vi "GeoData.vi"() -> ()   [LabVIEW 2017] (continued)
98357\t53009\tNeah bay\tWA\tClallam County\tH1\n98331\t53009\tForks\tWA\tClallam County\tH1\n98362\t53009\tPort angeles\tWA\tClallam County\tH1\n98343\t53009\tJoyce\tWA\tClallam County\tH1\n98350\t53009\tLa push\tWA\tClallam County\tH1\n98606\t53011\tBrush prairie\tWA\tClark County\tH1\n98601\t53011\tAmboy\tWA\tClark County\tH1\n98671\t53011\tWashougal\tWA\tClark County\tH1\n98674\t53011\tWoodland\tWA\tClark County\tH1\n98682\t53011\tVancouver\tWA\tClark County\tH1\n98668\t53011\tVancouver\tWA\tClark County\tH1\n98607\t53011\tCamas\tWA\tClark County\tH1\n98662\t53011\tVancouver\tWA\tClark County\tH1\n98687\t53011\tVancouver\tWA\tClark County\tH1\n98604\t53011\tBattle ground\tWA\tClark County\tH1\n98642\t53011\tRidgefield\tWA\tClark County\tH1\n98629\t53011\tLa center\tWA\tClark County\tH1\n98663\t53011\tVancouver\tWA\tClark County\tH1\n98685\t53011\tVancouver\tWA\tClark County\tH1\n98622\t53011\tHeisson\tWA\tClark County\tH1\n98664\t53011\tVancouver\tWA\tClark County\tH1\n98686\t53011\tVancouver\tWA\tClark County\tH1\n98660\t53011\tVancouver\tWA\tClark County\tH1\n98683\t53011\tVancouver\tWA\tClark County\tH1\n98665\t53011\tVancouver\tWA\tClark County\tH1\n98684\t53011\tVancouver\tWA\tClark County\tH1\n98675\t53011\tYacolt\tWA\tClark County\tH1\n98666\t53011\tVancouver\tWA\tClark County\tH1\n98661\t53011\tVancouver\tWA\tClark County\tH1\n99328\t53013\tDayton\tWA\tColumbia County\tH1\n99361\t53013\tWaitsburg\tWA\tColumbia County\tH1\n99359\t53013\tStarbuck\tWA\tColumbia County\tH1\n99347\t53013\tPomeroy\tWA\tColumbia County\tH1\n99348\t53013\tPrescott\tWA\tColumbia County\tH1\n99143\t53013\tLacrosse\tWA\tColumbia County\tH1\n98601\t53015\tAmboy\tWA\tCowlitz County\tH1\n98674\t53015\tWoodland\tWA\tCowlitz County\tH1\n98581\t53015\tRyderwood\tWA\tCowlitz County\tH1\n98609\t53015\tCarrolls\tWA\tCowlitz County\tH1\n98649\t53015\tToutle\tWA\tCowlitz County\tH1\n98611\t53015\tCastle rock\tWA\tCowlitz County\tH1\n98625\t53015\tKalama\tWA\tCowlitz County\tH1\n98645\t53015\tSilverlake\tWA\tCowlitz County\tH1\n98616\t53015\tCougar\tWA\tCowlitz County\tH1\n98632\t53015\tLongview\tWA\tCowlitz County\tH1\n98603\t53015\tAriel\tWA\tCowlitz County\tH1\n98626\t53015\tKelso\tWA\tCowlitz County\tH1\n98858\t53017\tWaterville\tWA\tDouglas County\tH1\n98845\t53017\tPalisades\tWA\tDouglas County\tH1\n98848\t53017\tQuincy\tWA\tDouglas County\tH1\n98830\t53017\tMansfield\tWA\tDouglas County\tH1\n98802\t53017\tEast wenatchee\tWA\tDouglas County\tH1\n99133\t53017\tGrand coulee\tWA\tDouglas County\tH1\n98823\t53017\tEphrata\tWA\tDouglas County\tH1\n98843\t53017\tOrondo\tWA\tDouglas County\tH1\n98850\t53017\tRock island\tWA\tDouglas County\tH1\n98812\t53017\tBrewster\tWA\tDouglas County\tH1\n99115\t53017\tCoulee city\tWA\tDouglas County\tH1\n99116\t53017\tCoulee dam\tWA\tDouglas County\tH1\n98813\t53017\tBridgeport\tWA\tDouglas County\tH1\n99121\t53019\tDanville\tWA\tFerry County\tH1\n99166\t53019\tRepublic\tWA\tFerry County\tH1\n99118\t53019\tCurlew\tWA\tFerry County\tH1\n99141\t53019\tKettle falls\tWA\tFerry County\tH1\n99146\t53019\tLaurier\tWA\tFerry County\tH1\n99140\t53019\tKeller\tWA\tFerry County\tH1\n99138\t53019\tInchelium\tWA\tFerry County\tH1\n99150\t53019\tMalo\tWA\tFerry County\tH1\n99160\t53019\tOrient\tWA\tFerry County\tH1\n99330\t53021\tEltopia\tWA\tFranklin County\tH1\n99371\t53021\tWashtucna\tWA\tFranklin County\tH1\n99335\t53021\tKahlotus\tWA\tFranklin County\tH1\n99343\t53021\tMesa\tWA\tFranklin County\tH1\n99344\t53021\tOthello\tWA\tFranklin County\tH1\n99302\t53021\tPasco\tWA\tFranklin County\tH1\n99301\t53021\tPasco\tWA\tFranklin County\tH1\n99326\t53021\tConnell\tWA\tFranklin County\tH1\n99328\t53023\tDayton\tWA\tGarfield County\tH1\n99347\t53023\tPomeroy\tWA\tGarfield County\tH1\n99403\t53023\tClarkston\tWA\tGarfield County\tH1\n98857\t53025\tWarden\tWA\tGrant County\tH1\n99357\t53025\tRoyal city\tWA\tGrant County\tH1\n98858\t53025\tWaterville\tWA\tGrant County\tH1\n98860\t53025\tWilson creek\tWA\tGrant County\tH1\n98851\t53025\tSoap lake\tWA\tGrant County\tH1\n99103\t53025\tAlmira\tWA\tGrant County\tH1\n98824\t53025\tGeorge\tWA\tGrant County\tH1\n98848\t53025\tQuincy\tWA\tGrant County\tH1\n99349\t53025\tMattawa\tWA\tGrant County\tH1\n98853\t53025\tStratford\tWA\tGrant County\tH1\n99133\t53025\tGrand coulee\tWA\tGrant County\tH1\n99123\t53025\tElectric city\tWA\tGrant County\tH1\n99344\t53025\tOthello\tWA\tGrant County\tH1\n99321\t53025\tBeverly\tWA\tGrant County\tH1\n98832\t53025\tMarlin\tWA\tGrant County\tH1\n98823\t53025\tEphrata\tWA\tGrant County\tH1\n99135\t53025\tHartline\tWA\tGrant County\tH1\n98837\t53025\tMoses lake\tWA\tGrant County\tH1\n99115\t53025\tCoulee city\tWA\tGrant County\tH1\n99116\t53025\tCoulee dam\tWA\tGrant County\tH1\n98537\t53027\tCosmopolis\tWA\tGrays Harbor County\tH1\n98563\t53027\tMontesano\tWA\tGrays Harbor County\tH1\n98595\t53027\tWestport\tWA\tGrays Harbor County\tH1\n98550\t53027\tHoquiam\tWA\tGrays Harbor County\tH1\n98583\t53027\tSatsop\tWA\tGrays Harbor County\tH1\n98569\t53027\tOcean shores\tWA\tGrays Harbor County\tH1\n98520\t53027\tAberdeen\tWA\tGrays Harbor County\tH1\n98526\t53027\tAmanda park\tWA\tGrays Harbor County\tH1\n98575\t53027\tQuinault\tWA\tGrays Harbor County\tH1\n98562\t53027\tMoclips\tWA\tGrays Harbor County\tH1\n98557\t53027\tMccleary\tWA\tGrays Harbor County\tH1\n98579\t53027\tRochester\tWA\tGrays Harbor County\tH1\n98541\t53027\tElma\tWA\tGrays Harbor County\tH1\n98547\t53027\tGrayland\tWA\tGrays Harbor County\tH1\n98568\t53027\tOakville\tWA\tGrays Harbor County\tH1\n98536\t53027\tCopalis crossing\tWA\tGrays Harbor County\tH1\n98566\t53027\tNeilton\tWA\tGrays Harbor County\tH1\n98535\t53027\tCopalis beach\tWA\tGrays Harbor County\tH1\n98571\t53027\tPacific beach\tWA\tGrays Harbor County\tH1\n98552\t53027\tHumptulips\tWA\tGrays Harbor County\tH1\n98559\t53027\tMalone\tWA\tGrays Harbor County\tH1\n98587\t53027\tTaholah\tWA\tGrays Harbor County\tH1\n98249\t53029\tFreeland\tWA\tIsland County\tH1\n98278\t53029\tOak harbor\tWA\tIsland County\tH1\n98277\t53029\tOak harbor\tWA\tIsland County\tH1\n98282\t53029\tCamano island\tWA\tIsland County\tH1\n98260\t53029\tLangley\tWA\tIsland County\tH1\n98236\t53029\tClinton\tWA\tIsland County\tH1\n98253\t53029\tGreenbank\tWA\tIsland County\tH1\n98239\t53029\tCoupeville\tWA\tIsland County\tH1\n98320\t53031\tBrinnon\tWA\tJefferson County\tH1\n98376\t53031\tQuilcene\tWA\tJefferson County\tH1\n98368\t53031\tPort townsend\tWA\tJefferson County\tH1\n98365\t53031\tPort ludlow\tWA\tJefferson County\tH1\n98382\t53031\tSequim\tWA\tJefferson County\tH1\n98331\t53031\tForks\tWA\tJefferson County\tH1\n98339\t53031\tPort hadlock\tWA\tJefferson County\tH1\n98325\t53031\tChimacum\tWA\tJefferson County\tH1\n98358\t53031\tNordland\tWA\tJefferson County\tH1\n98102\t53033\tSeattle\tWA\tKing County\tH1\n98103\t53033\tSeattle\tWA\tKing County\tH1\n98115\t53033\tSeattle\tWA\tKing County\tH1\n98058\t53033\tRenton\tWA\tKing County\tH1\n98070\t53033\tVashon\tWA\tKing County\tH1\n98122\t53033\tSeattle\tWA\tKing County\tH1\n98083\t53033\tKirkland\tWA\tKing County\tH1\n98111\t53033\tSeattle\tWA\tKing County\tH1\n98198\t53033\tSeattle\tWA\tKing County\tH1\n98133\t53033\tSeattle\tWA\tKing County\tH1\n98136\t53033\tSeattle\tWA\tKing County\tH1\n98134\t53033\tSeattle\tWA\tKing County\tH1\n98034\t53033\tKirkland\tWA\tKing County\tH1\n98023\t53033\tFederal way\tWA\tKing County\tH1\n98052\t53033\tRedmond\tWA\tKing County\tH1\n98021\t53033\tBothell\tWA\tKing County\tH1\n98055\t53033\tRenton\tWA\tKing County\tH1\n98051\t53033\tRavensdale\tWA\tKing County\tH1\n98194\t53033\tSeattle\tWA\tKing County\tH1\n98175\t53033\tSeattle\tWA\tKing County\tH1\n98224\t53033\tBaring\tWA\tKing County\tH1\n98004\t53033\tBellevue\tWA\tKing County\tH1\n98007\t53033\tBellevue\tWA\tKing County\tH1\n98008\t53033\tBellevue\tWA\tKing County\tH1\n98019\t53033\tDuvall\tWA\tKing County\tH1\n98014\t53033\tCarnation\tWA\tKing County\tH1\n98092\t53033\tAuburn\tWA\tKing County\tH1\n98074\t53033\tSammamish\tWA\tKing County\tH1\n98106\t53033\tSeattle\tWA\tKing County\tH1\n98354\t53033\tMilton\tWA\tKing County\tH1\n98030\t53033\tKent\tWA\tKing County\tH1\n98288\t53033\tSkykomish\tWA\tKing County\tH1\n98035\t53033\tKent\tWA\tKing County\tH1\n98131\t53033\tSeattle\tWA\tKing County\tH1\n98001\t53033\tAuburn\tWA\tKing County\tH1\n98119\t53033\tSeattle\tWA\tKing County\tH1\n98144\t53033\tSeattle\tWA\tKing County\tH1\n98126\t53033\tSeattle\tWA\tKing County\tH1\n98124\t53033\tSeattle\tWA\tKing County\tH1\n98042\t53033\tKent\tWA\tKing County\tH1\n98158\t53033\tSeattle\tWA\tKing County\tH1\n98073\t53033\tRedmond\tWA\tKing County\tH1\n98113\t53033\tSeattle\tWA\tKing County\tH1\n98071\t53033\tAuburn\tWA\tKing County\tH1\n98062\t53033\tSeahurst\tWA\tKing County\tH1\n98129\t53033\tSeattle\tWA\tKing County\tH1\n98002\t53033\tAuburn\tWA\tKing County\tH1\n98011\t53033\tBothell\tWA\tKing County\tH1\n98006\t53033\tBellevue\tWA\tKing County\tH1\n98188\t53033\tSeattle\tWA\tKing County\tH1\n98199\t53033\tSeattle\tWA\tKing County\tH1\n98031\t53033\tKent\tWA\tKing County\tH1\n98022\t53033\tEnumclaw\tWA\tKing County\tH1\n98033\t53033\tKirkland\tWA\tKing County\tH1\n98039\t53033\tMedina\tWA\tKing County\tH1\n98057\t53033\tRenton\tWA\tKing County\tH1\n98045\t53033\tNorth bend\tWA\tKing County\tH1\n98089\t53033\tKent\tWA\tKing County\tH1\n98063\t53033\tFederal way\tWA\tKing County\tH1\n98025\t53033\tHobart\tWA\tKing County\tH1\n98191\t53033\tSeattle\tWA\tKing County\tH1\n98003\t53033\tFederal way\tWA\tKing County\tH1\n98109\t53033\tSeattle\tWA\tKing County\tH1\n98117\t53033\tSeattle\tWA\tKing County\tH1\n98118\t53033\tSeattle\tWA\tKing County\tH1\n98121\t53033\tSeattle\tWA\tKing County\tH1\n98155\t53033\tSeattle\tWA\tKing County\tH1\n98038\t53033\tMaple valley\tWA\tKing County\tH1\n98032\t53033\tKent\tWA\tKing County\tH1\n98024\t53033\tFall city\tWA\tKing County\tH1\n98053\t53033\tRedmond\tWA\tKing County\tH1\n98138\t53033\tSeattle\tWA\tKing County\tH1\n98181\t53033\tSeattle\tWA\tKing County\tH1\n98010\t53033\tBlack diamond\tWA\tKing County\tH1\n98107\t53033\tSeattle\tWA\tKing County\tH1\n98065\t53033\tSnoqualmie\tWA\tKing County\tH1\n98072\t53033\tWoodinville\tWA\tKing County\tH1\n98112\t53033\tSeattle\tWA\tKing County\tH1\n98146\t53033\tSeattle\tWA\tKing County\tH1\n98148\t53033\tSeattle\tWA\tKing County\tH1\n98145\t53033\tSeattle\tWA\tKing County\tH1\n98185\t53033\tSeattle\tWA\tKing County\tH1\n98050\t53033\tPreston\tWA\tKing County\tH1\n98009\t53033\tBellevue\tWA\tKing County\tH1\n98101\t53033\tSeattle\tWA\tKing County\tH1\n98108\t53033\tSeattle\tWA\tKing County\tH1\n98077\t53033\tWoodinville\tWA\tKing County\tH1\n98093\t53033\tFederal way\tWA\tKing County\tH1\n98251\t53033\tGold bar\tWA\tKing County\tH1\n98422\t53033\tTacoma\tWA\tKing County\tH1\n98168\t53033\tSeattle\tWA\tKing County\tH1\n98177\t53033\tSeattle\tWA\tKing County\tH1\n98125\t53033\tSeattle\tWA\tKing County\tH1\n98178\t53033\tSeattle\tWA\tKing County\tH1\n98127\t53033\tSeattle\tWA\tKing County\tH1\n98028\t53033\tKenmore\tWA\tKing County\tH1\n98047\t53033\tPacific\tWA\tKing County\tH1\n98164\t53033\tSeattle\tWA\tKing County\tH1\n98015\t53033\tBellevue\tWA\tKing County\tH1\n98154\t53033\tSeattle\tWA\tKing County\tH1\n98195\t53033\tSeattle\tWA\tKing County\tH1\n98068\t53033\tSnoqualmie pass\tWA\tKing County\tH1\n98005\t53033\tBellevue\tWA\tKing County\tH1\n98104\t53033\tSeattle\tWA\tKing County\tH1\n98105\t53033\tSeattle\tWA\tKing County\tH1\n98059\t53033\tRenton\tWA\tKing County\tH1\n98075\t53033\tSammamish\tWA\tKing County\tH1\n98116\t53033\tSeattle\tWA\tKing County\tH1\n98166\t53033\tSeattle\tWA\tKing County\tH1\n98029\t53033\tIssaquah\tWA\tKing County\tH1\n98040\t53033\tMercer island\tWA\tKing County\tH1\n98027\t53033\tIssaquah\tWA\tKing County\tH1\n98056\t53033\tRenton\tWA\tKing County\tH1\n98165\t53033\tSeattle\tWA\tKing County\tH1\n98041\t53033\tBothell\tWA\tKing County\tH1\n98139\t53033\tSeattle\tWA\tKing County\tH1\n98174\t53033\tSeattle\tWA\tKing County\tH1\n98064\t53033\tKent\tWA\tKing County\tH1\n98161\t53033\tSeattle\tWA\tKing County\tH1\n98114\t53033\tSeattle\tWA\tKing County\tH1\n98359\t53035\tOlalla\tWA\tKitsap County\tH1\n98353\t53035\tManchester\tWA\tKitsap County\tH1\n98312\t53035\tBremerton\tWA\tKitsap County\tH1\n98329\t53035\tGig harbor\tWA\tKitsap County\tH1\n98380\t53035\tSeabeck\tWA\tKitsap County\tH1\n98342\t53035\tIndianola\tWA\tKitsap County\tH1\n98340\t53035\tHansville\tWA\tKitsap County\tH1\n98364\t53035\tPort gamble\tWA\tKitsap County\tH1\n98366\t53035\tPort orchard\tWA\tKitsap County\tH1\n98110\t53035\tBainbridge island\tWA\tKitsap County\tH1\n98370\t53035\tPoulsbo\tWA\tKitsap County\tH1\n98346\t53035\tKingston\tWA\tKitsap County\tH1\n98322\t53035\tBurley\tWA\tKitsap County\tH1\n98384\t53035\tSouth colby\tWA\tKitsap County\tH1\n98315\t53035\tSilverdale\tWA\tKitsap County\tH1\n98392\t53035\tSuquamish\tWA\tKitsap County\tH1\n98393\t53035\tTracyton\tWA\tKitsap County\tH1\n98345\t53035\tKeyport\tWA\tKitsap County\tH1\n98061\t53035\tRollingbay\tWA\tKitsap County\tH1\n98311\t53035\tBremerton\tWA\tKitsap County\tH1\n98310\t53035\tBremerton\tWA\tKitsap County\tH1\n98367\t53035\tPort orchard\tWA\tKitsap County\tH1\n98337\t53035\tBremerton\tWA\tKitsap County\tH1\n98314\t53035\tBremerton\tWA\tKitsap County\tH1\n98383\t53035\tSilverdale\tWA\tKitsap County\tH1\n98528\t53035\tBelfair\tWA\tKitsap County\tH1\n98386\t53035\tSouthworth\tWA\tKitsap County\tH1\n98828\t53037\tMalaga\tWA\tKittitas County\tH1\n98941\t53037\tRoslyn\tWA\tKittitas County\tH1\n98922\t53037\tCle elum\tWA\tKittitas County\tH1\n98926\t53037\tEllensburg\tWA\tKittitas County\tH1\n98943\t53037\tSouth cle elum\tWA\tKittitas County\tH1\n98950\t53037\tVantage\tWA\tKittitas County\tH1\n98901\t53037\tYakima\tWA\tKittitas County\tH1\n98946\t53037\tThorp\tWA\tKittitas County\tH1\n98925\t53037\tEaston\tWA\tKittitas County\tH1\n98812\t53037\tBrewster\tWA\tKittitas County\tH1\n98940\t53037\tRonald\tWA\tKittitas County\tH1\n98068\t53037\tSnoqualmie pass\tWA\tKittitas County\tH1\n98934\t53037\tKittitas\tWA\tKittitas County\tH1\n98623\t53039\tHusum\tWA\tKlickitat County\tH1\n98617\t53039\tDallesport\tWA\tKlickitat County\tH1\n99356\t53039\tRoosevelt\tWA\tKlickitat County\tH1\n99322\t53039\tBickleton\tWA\tKlickitat County\tH1\n98620\t53039\tGoldendale\tWA\tKlickitat County\tH1\n98605\t53039\tBingen\tWA\tKlickitat County\tH1\n98673\t53039\tWishram\tWA\tKlickitat County\tH1\n98650\t53039\tTrout lake\tWA\tKlickitat County\tH1\n98635\t53039\tLyle\tWA\tKlickitat County\tH1\n99350\t53039\tProsser\tWA\tKlickitat County\tH1\n98602\t53039\tAppleton\tWA\tKlickitat County\tH1\n98935\t53039\tMabton\tWA\tKlickitat County\tH1\n98651\t53039\tUnderwood\tWA\tKlickitat County\tH1\n98619\t53039\tGlenwood\tWA\tKlickitat County\tH1\n98628\t53039\tKlickitat\tWA\tKlickitat County\tH1\n98672\t53039\tWhite salmon\tWA\tKlickitat County\tH1\n98613\t53039\tCenterville\tWA\tKlickitat County\tH1\n98670\t53039\tWahkiacus\tWA\tKlickitat County\tH1\n98539\t53041\tDoty\tWA\tLewis County\tH1\n98330\t53041\tElbe\tWA\tLewis County\tH1\n98355\t53041\tMineral\tWA\tLewis County\tH1\n98532\t53041\tChehalis\tWA\tLewis County\tH1\n98572\t53041\tPe ell\tWA\tLewis County\tH1\n98538\t53041\tCurtis\tWA\tLewis County\tH1\n98582\t53041\tSalkum\tWA\tLewis County\tH1\n98377\t53041\tRandle\tWA\tLewis County\tH1\n98533\t53041\tCinebar\tWA\tLewis County\tH1\n98579\t53041\tRochester\tWA\tLewis County\tH1\n98591\t53041\tToledo\tWA\tLewis County\tH1\n98542\t53041\tEthel\tWA\tLewis County\tH1\n98304\t53041\tAshford\tWA\tLewis County\tH1\n98531\t53041\tCentralia\tWA\tLewis County\tH1\n98596\t53041\tWinlock\tWA\tLewis County\tH1\n98361\t53041\tPackwood\tWA\tLewis County\tH1\n98593\t53041\tVader\tWA\tLewis County\tH1\n98522\t53041\tAdna\tWA\tLewis County\tH1\n98544\t53041\tGalvin\tWA\tLewis County\tH1\n98570\t53041\tOnalaska\tWA\tLewis County\tH1\n98568\t53041\tOakville\tWA\tLewis County\tH1\n98585\t53041\tSilver creek\tWA\tLewis County\tH1\n98336\t53041\tGlenoma\tWA\tLewis County\tH1\n98356\t53041\tMorton\tWA\tLewis County\tH1\n98564\t53041\tMossyrock\tWA\tLewis County\tH1\n98565\t53041\tNapavine\tWA\tLewis County\tH1\n99032\t53043\tSprague\tWA\tLincoln County\tH1\n99154\t53043\tMohler\tWA\tLincoln County\tH1\n99144\t53043\tLamona\tWA\tLincoln County\tH1\n99185\t53043\tWilbur\tWA\tLincoln County\tH1\n99103\t53043\tAlmira\tWA\tLincoln County\tH1\n99147\t53043\tLincoln\tWA\tLincoln County\tH1\n99169\t53043\tRitzville\tWA\tLincoln County\tH1\n99133\t53043\tGrand coulee\tWA\tLincoln County\tH1\n99029\t53043\tReardan\tWA\tLincoln County\tH1\n99134\t53043\tHarrington\tWA\tLincoln County\tH1\n99122\t53043\tDavenport\tWA\tLincoln County\tH1\n98832\t53043\tMarlin\tWA\tLincoln County\tH1\n99008\t53043\tEdwall\tWA\tLincoln County\tH1\n99159\t53043\tOdessa\tWA\tLincoln County\tH1\n99117\t53043\tCreston\tWA\tLincoln County\tH1\n99013\t53043\tFord\tWA\tLincoln County\tH1\n98563\t53045\tMontesano\tWA\tMason County\tH1\n98312\t53045\tBremerton\tWA\tMason County\tH1\n98380\t53045\tSeabeck\tWA\tMason County\tH1\n98592\t53045\tUnion\tWA\tMason County\tH1\n98560\t53045\tMatlock\tWA\tMason County\tH1\n98502\t53045\tOlympia\tWA\tMason County\tH1\n98557\t53045\tMccleary\tWA\tMason County\tH1\n98524\t53045\tAllyn\tWA\tMason County\tH1\n98541\t53045\tElma\tWA\tMason County\tH1\n98584\t53045\tShelton\tWA\tMason County\tH1\n98588\t53045\tTahuya\tWA\tMason County\tH1\n98555\t53045\tLilliwaup\tWA\tMason County\tH1\n98548\t53045\tHoodsport\tWA\tMason County\tH1\n98528\t53045\tBelfair\tWA\tMason County\tH1\n98546\t53045\tGrapeview\tWA\tMason County\tH1\n98862\t53047\tWinthrop\tWA\tOkanogan County\tH1\n99124\t53047\tElmer city\tWA\tOkanogan County\tH1\n98816\t53047\tChelan\tWA\tOkanogan County\tH1\n98814\t53047\tCarlton\tWA\tOkanogan County\tH1\n99166\t53047\tRepublic\tWA\tOkanogan County\tH1\n98846\t53047\tPateros\tWA\tOkanogan County\tH1\n98819\t53047\tConconully\tWA\tOkanogan County\tH1\n98849\t53047\tRiverside\tWA\tOkanogan County\tH1\n98834\t53047\tMethow\tWA\tOkanogan County\tH1\n98844\t53047\tOroville\tWA\tOkanogan County\tH1\n99133\t53047\tGrand coulee\tWA\tOkanogan County\tH1\n98841\t53047\tOmak\tWA\tOkanogan County\tH1\n98833\t53047\tMazama\tWA\tOkanogan County\tH1\n98855\t53047\tTonasket\tWA\tOkanogan County\tH1\n98840\t53047\tOkanogan\tWA\tOkanogan County\tH1\n98812\t53047\tBrewster\tWA\tOkanogan County\tH1\n98859\t53047\tWauconda\tWA\tOkanogan County\tH1\n98856\t53047\tTwisp\tWA\tOkanogan County\tH1\n99155\t53047\tNespelem\tWA\tOkanogan County\tH1\n98827\t53047\tLoomis\tWA\tOkanogan County\tH1\n99116\t53047\tCoulee dam\tWA\tOkanogan County\tH1\n98813\t53047\tBridgeport\tWA\tOkanogan County\tH1\n98829\t53047\tMalott\tWA\tOkanogan County\tH1\n98614\t53049\tChinook\tWA\tPacific County\tH1\n98624\t53049\tIlwaco\tWA\tPacific County\tH1\n98537\t53049\tCosmopolis\tWA\tPacific County\tH1\n98641\t53049\tOysterville\tWA\tPacific County\tH1\n98561\t53049\tMenlo\tWA\tPacific County\tH1\n98640\t53049\tOcean park\tWA\tPacific County\tH1\n98644\t53049\tSeaview\tWA\tPacific County\tH1\n98554\t53049\tLebam\tWA\tPacific County\tH1\n98572\t53049\tPe ell\tWA\tPacific County\tH1\n98527\t53049\tBay center\tWA\tPacific County\tH1\n98586\t53049\tSouth bend\tWA\tPacific County\tH1\n98590\t53049\tTokeland\tWA\tPacific County\tH1\n98637\t53049\tNahcotta\tWA\tPacific County\tH1\n98631\t53049\tLong beach\tWA\tPacific County\tH1\n98547\t53049\tGrayland\tWA\tPacific County\tH1\n98638\t53049\tNaselle\tWA\tPacific County\tH1\n98577\t53049\tRaymond\tWA\tPacific County\tH1\n99006\t53051\tDeer park\tWA\tPend Oreille County\tH1\n99009\t53051\tElk\tWA\tPend Oreille County\tH1\n99156\t53051\tNewport\tWA\tPend Oreille County\tH1\n99180\t53051\tUsk\tWA\tPend Oreille County\tH1\n99139\t53051\tIone\tWA\tPend Oreille County\tH1\n99153\t53051\tMetaline falls\tWA\tPend Oreille County\tH1\n99119\t53051\tCusick\tWA\tPend Oreille County\tH1\n99152\t53051\tMetaline\tWA\tPend Oreille County\tH1\n98328\t53053\tEatonville\tWA\tPierce County\tH1\n98372\t53053\tPuyallup\tWA\tPierce County\tH1\n98391\t53053\tBonney lake\tWA\tPierce County\tH1\n98359\t53053\tOlalla\tWA\tPierce County\tH1\n98409\t53053\tTacoma\tWA\tPierce County\tH1\n98424\t53053\tTacoma\tWA\tPierce County\tH1\n98408\t53053\tTacoma\tWA\tPierce County\tH1\n98023\t53053\tFederal way\tWA\tPierce County\tH1\n98419\t53053\tTacoma\tWA\tPierce County\tH1\n98092\t53053\tAuburn\tWA\tPierce County\tH1\n98321\t53053\tBuckley\tWA\tPierce County\tH1\n98329\t53053\tGig harbor\tWA\tPierce County\tH1\n98332\t53053\tGig harbor\tWA\tPierce County\tH1\n98360\t53053\tOrting\tWA\tPierce County\tH1\n98354\t53053\tMilton\tWA\tPierce County\tH1\n98385\t53053\tSouth prairie\tWA\tPierce County\tH1\n98416\t53053\tTacoma\tWA\tPierce County\tH1\n98580\t53053\tRoy\tWA\tPierce County\tH1\n98464\t53053\tTacoma\tWA\tPierce County\tH1\n98496\t53053\tLakewood\tWA\tPierce County\tH1\n98330\t53053\tElbe\tWA\tPierce County\tH1\n98327\t53053\tDupont\tWA\tPierce County\tH1\n98499\t53053\tLakewood\tWA\tPierce County\tH1\n98438\t53053\tMcchord afb\tWA\tPierce County\tH1\n98493\t53053\tTacoma\tWA\tPierce County\tH1\n98397\t53053\tLongmire\tWA\tPierce County\tH1\n98348\t53053\tLa grande\tWA\tPierce County\tH1\n98387\t53053\tSpanaway\tWA\tPierce County\tH1\n98338\t53053\tGraham\tWA\tPierce County\tH1\n98402\t53053\tTacoma\tWA\tPierce County\tH1\n98349\t53053\tLakebay\tWA\tPierce County\tH1\n98407\t53053\tTacoma\tWA\tPierce County\tH1\n98388\t53053\tSteilacoom\tWA\tPierce County\tH1\n98351\t53053\tLongbranch\tWA\tPierce County\tH1\n98446\t53053\tTacoma\tWA\tPierce County\tH1\n98443\t53053\tTacoma\tWA\tPierce County\tH1\n98418\t53053\tTacoma\tWA\tPierce County\tH1\n98498\t53053\tLakewood\tWA\tPierce County\tH1\n98022\t53053\tEnumclaw\tWA\tPierce County\tH1\n98421\t53053\tTacoma\tWA\tPierce County\tH1\n98371\t53053\tPuyallup\tWA\tPierce County\tH1\n98373\t53053\tPuyallup\tWA\tPierce County\tH1\n98374\t53053\tPuyallup\tWA\tPierce County\tH1\n98445\t53053\tTacoma\tWA\tPierce County\tH1\n98448\t53053\tTacoma\tWA\tPierce County\tH1\n98439\t53053\tLakewood\tWA\tPierce County\tH1\n98430\t53053\tCamp murray\tWA\tPierce County\tH1\n98417\t53053\tTacoma\tWA\tPierce County\tH1\n98558\t53053\tMckenna\tWA\tPierce County\tH1\n98395\t53053\tWauna\tWA\tPierce County\tH1\n98304\t53053\tAshford\tWA\tPierce County\tH1\n98323\t53053\tCarbonado\tWA\tPierce County\tH1\n98375\t53053\tPuyallup\tWA\tPierce County\tH1\n98394\t53053\tVaughn\tWA\tPierce County\tH1\n98467\t53053\tUniversity place\tWA\tPierce County\tH1\n98937\t53053\tNaches\tWA\tPierce County\tH1\n98433\t53053\tTacoma\tWA\tPierce County\tH1\n98490\t53053\tTacoma\tWA\tPierce County\tH1\n98344\t53053\tKapowsin\tWA\tPierce County\tH1\n98333\t53053\tFox island\tWA\tPierce County\tH1\n98404\t53053\tTacoma\tWA\tPierce County\tH1\n98405\t53053\tTacoma\tWA\tPierce County\tH1\n98422\t53053\tTacoma\tWA\tPierce County\tH1\n98047\t53053\tPacific\tWA\tPierce County\tH1\n98411\t53053\tTacoma\tWA\tPierce County\tH1\n98447\t53053\tTacoma\tWA\tPierce County\tH1\n98352\t53053\tSumner\tWA\tPierce County\tH1\n98335\t53053\tGig harbor\tWA\tPierce County\tH1\n98406\t53053\tTacoma\tWA\tPierce County\tH1\n98403\t53053\tTacoma\tWA\tPierce County\tH1\n98390\t53053\tSumner\tWA\tPierce County\tH1\n98444\t53053\tTacoma\tWA\tPierce County\tH1\n98466\t53053\tTacoma\tWA\tPierce County\tH1\n98465\t53053\tTacoma\tWA\tPierce County\tH1\n98528\t53053\tBelfair\tWA\tPierce County\tH1\n98303\t53053\tAnderson island\tWA\tPierce County\tH1\n98401\t53053\tTacoma\tWA\tPierce County\tH1\n98413\t53053\tTacoma\tWA\tPierce County\tH1\n98396\t53053\tWilkeson\tWA\tPierce County\tH1\n98398\t53053\tParadise inn\tWA\tPierce County\tH1\n98431\t53053\tTacoma\tWA\tPierce County\tH1\n98286\t53055\tShaw island\tWA\tSan Juan County\tH1\n98245\t53055\tEastsound\tWA\tSan Juan County\tH1\n98279\t53055\tOlga\tWA\tSan Juan County\tH1\n98261\t53055\tLopez island\tWA\tSan Juan County\tH1\n98222\t53055\tBlakely island\tWA\tSan Juan County\tH1\n98243\t53055\tDeer harbor\tWA\tSan Juan County\tH1\n98250\t53055\tFriday harbor\tWA\tSan Juan County\tH1\n98280\t53055\tOrcas\tWA\tSan Juan County\tH1\n98297\t53055\tWaldron\tWA\tSan Juan County\tH1\n98221\t53055\tAnacortes\tWA\tSan Juan County\tH1\n98274\t53057\tMount vernon\tWA\tSkagit County\tH1\n98267\t53057\tMarblemount\tWA\tSkagit County\tH1\n98233\t53057\tBurlington\tWA\tSkagit County\tH1\n98263\t53057\tLyman\tWA\tSkagit County\tH1\n98273\t53057\tMount vernon\tWA\tSkagit County\tH1\n98237\t53057\tConcrete\tWA\tSkagit County\tH1\n98257\t53057\tLa conner\tWA\tSkagit County\tH1\n98235\t53057\tClearlake\tWA\tSkagit County\tH1\n98284\t53057\tSedro woolley\tWA\tSkagit County\tH1\n98232\t53057\tBow\tWA\tSkagit County\tH1\n98283\t53057\tRockport\tWA\tSkagit County\tH1\n98241\t53057\tDarrington\tWA\tSkagit County\tH1\n98221\t53057\tAnacortes\tWA\tSkagit County\tH1\n98255\t53057\tHamilton\tWA\tSkagit County\tH1\n98292\t53057\tStanwood\tWA\tSkagit County\tH1\n98229\t53057\tBellingham\tWA\tSkagit County\tH1\n98238\t53057\tConway\tWA\tSkagit County\tH1\n98671\t53059\tWashougal\tWA\tSkamania County\tH1\n98610\t53059\tCarson\tWA\tSkamania County\tH1\n98605\t53059\tBingen\tWA\tSkamania County\tH1\n98639\t53059\tNorth bonneville\tWA\tSkamania County\tH1\n98616\t53059\tCougar\tWA\tSkamania County\tH1\n98651\t53059\tUnderwood\tWA\tSkamania County\tH1\n98672\t53059\tWhite salmon\tWA\tSkamania County\tH1\n98648\t53059\tStevenson\tWA\tSkamania County\tH1\n98270\t53061\tMarysville\tWA\tSnohomish County\tH1\n98213\t53061\tEverett\tWA\tSnohomish County\tH1\n98037\t53061\tLynnwood\tWA\tSnohomish County\tH1\n98021\t53061\tBothell\tWA\tSnohomish County\tH1\n98291\t53061\tSnohomish\tWA\tSnohomish County\tH1\n98019\t53061\tDuvall\tWA\tSnohomish County\tH1\n98087\t53061\tLynnwood\tWA\tSnohomish County\tH1\n98296\t53061\tSnohomish\tWA\tSnohomish County\tH1\n98223\t53061\tArlington\tWA\tSnohomish County\tH1\n98272\t53061\tMonroe\tWA\tSnohomish County\tH1\n98282\t53061\tCamano island\tWA\tSnohomish County\tH1\n98287\t53061\tSilvana\tWA\tSnohomish County\tH1\n98294\t53061\tSultan\tWA\tSnohomish County\tH1\n98011\t53061\tBothell\tWA\tSnohomish County\tH1\n98275\t53061\tMukilteo\tWA\tSnohomish County\tH1\n98290\t53061\tSnohomish\tWA\tSnohomish County\tH1\n98271\t53061\tMarysville\tWA\tSnohomish County\tH1\n98206\t53061\tEverett\tWA\tSnohomish County\tH1\n98207\t53061\tEverett\tWA\tSnohomish County\tH1\n98258\t53061\tLake stevens\tWA\tSnohomish County\tH1\n98204\t53061\tEverett\tWA\tSnohomish County\tH1\n98020\t53061\tEdmonds\tWA\tSnohomish County\tH1\n98082\t53061\tMill creek\tWA\tSnohomish County\tH1\n98046\t53061\tLynnwood\tWA\tSnohomish County\tH1\n98072\t53061\tWoodinville\tWA\tSnohomish County\tH1\n98203\t53061\tEverett\tWA\tSnohomish County\tH1\n98043\t53061\tMountlake terrace\tWA\tSnohomish County\tH1\n98012\t53061\tBothell\tWA\tSnohomish County\tH1\n98077\t53061\tWoodinville\tWA\tSnohomish County\tH1\n98251\t53061\tGold bar\tWA\tSnohomish County\tH1\n98241\t53061\tDarrington\tWA\tSnohomish County\tH1\n98177\t53061\tSeattle\tWA\tSnohomish County\tH1\n98208\t53061\tEverett\tWA\tSnohomish County\tH1\n98028\t53061\tKenmore\tWA\tSnohomish County\tH1\n98292\t53061\tStanwood\tWA\tSnohomish County\tH1\n98252\t53061\tGranite falls\tWA\tSnohomish County\tH1\n98201\t53061\tEverett\tWA\tSnohomish County\tH1\n98036\t53061\tLynnwood\tWA\tSnohomish County\tH1\n98026\t53061\tEdmonds\tWA\tSnohomish County\tH1\n98259\t53061\tNorth lakewood\tWA\tSnohomish County\tH1\n98293\t53061\tStartup\tWA\tSnohomish County\tH1\n98256\t53061\tIndex\tWA\tSnohomish County\tH1\n99006\t53063\tDeer park\tWA\tSpokane County\tH1\n99023\t53063\tMica\tWA\tSpokane County\tH1\n99025\t53063\tNewman lake\tWA\tSpokane County\tH1\n99036\t53063\tValleyford\tWA\tSpokane County\tH1\n99209\t53063\tSpokane\tWA\tSpokane County\tH1\n99170\t53063\tRosalia\tWA\tSpokane County\tH1\n99228\t53063\tSpokane\tWA\tSpokane County\tH1\n99032\t53063\tSprague\tWA\tSpokane County\tH1\n99210\t53063\tSpokane\tWA\tSpokane County\tH1\n99211\t53063\tSpokane\tWA\tSpokane County\tH1\n99018\t53063\tLatah\tWA\tSpokane County\tH1\n99260\t53063\tSpokane\tWA\tSpokane County\tH1\n99009\t53063\tElk\tWA\tSpokane County\tH1\n99212\t53063\tSpokane\tWA\tSpokane County\tH1\n99027\t53063\tOtis orchards\tWA\tSpokane County\tH1\n99033\t53063\tTekoa\tWA\tSpokane County\tH1\n99219\t53063\tSpokane\tWA\tSpokane County\tH1\n99003\t53063\tChattaroy\tWA\tSpokane County\tH1\n99004\t53063\tCheney\tWA\tSpokane County\tH1\n99037\t53063\tVeradale\tWA\tSpokane County\tH1\n99203\t53063\tSpokane\tWA\tSpokane County\tH1\n99026\t53063\tNine mile falls\tWA\tSpokane County\tH1\n99031\t53063\tSpangle\tWA\tSpokane County\tH1\n99020\t53063\tMarshall\tWA\tSpokane County\tH1\n99016\t53063\tGreenacres\tWA\tSpokane County\tH1\n99201\t53063\tSpokane\tWA\tSpokane County\tH1\n99202\t53063\tSpokane\tWA\tSpokane County\tH1\n99205\t53063\tSpokane\tWA\tSpokane County\tH1\n99156\t53063\tNewport\tWA\tSpokane County\tH1\n99030\t53063\tRockford\tWA\tSpokane County\tH1\n99218\t53063\tSpokane\tWA\tSpokane County\tH1\n99204\t53063\tSpokane\tWA\tSpokane County\tH1\n99214\t53063\tSpokane\tWA\tSpokane County\tH1\n99258\t53063\tSpokane\tWA\tSpokane County\tH1\n99252\t53063\tSpokane\tWA\tSpokane County\tH1\n99019\t53063\tLiberty lake\tWA\tSpokane County\tH1\n99012\t53063\tFairfield\tWA\tSpokane County\tH1\n99206\t53063\tSpokane\tWA\tSpokane County\tH1\n99217\t53063\tSpokane\tWA\tSpokane County\tH1\n99029\t53063\tReardan\tWA\tSpokane County\tH1\n99213\t53063\tSpokane\tWA\tSpokane County\tH1\n99001\t53063\tAirway heights\tWA\tSpokane County\tH1\n99207\t53063\tSpokane\tWA\tSpokane County\tH1\n99208\t53063\tSpokane\tWA\tSpokane County\tH1\n99216\t53063\tSpokane\tWA\tSpokane County\tH1\n99220\t53063\tSpokane\tWA\tSpokane County\tH1\n99256\t53063\tSpokane\tWA\tSpokane County\tH1\n99014\t53063\tFour lakes\tWA\tSpokane County\tH1\n99251\t53063\tSpokane\tWA\tSpokane County\tH1\n99005\t53063\tColbert\tWA\tSpokane County\tH1\n99021\t53063\tMead\tWA\tSpokane County\tH1\n99110\t53063\tClayton\tWA\tSpokane County\tH1\n99008\t53063\tEdwall\tWA\tSpokane County\tH1\n99022\t53063\tMedical lake\tWA\tSpokane County\tH1\n99223\t53063\tSpokane\tWA\tSpokane County\tH1\n99224\t53063\tSpokane\tWA\tSpokane County\tH1\n99011\t53063\tFairchild air force base\tWA\tSpokane County\tH1\n99013\t53063\tFord\tWA\tSpokane County\tH1\n99039\t53063\tWaverly\tWA\tSpokane County\tH1\n99006\t53065\tDeer park\tWA\tStevens County\tH1\n99109\t53065\tChewelah\tWA\tStevens County\tH1\n99034\t53065\tTumtum\tWA\tStevens County\tH1\n99157\t53065\tNorthport\tWA\tStevens County\tH1\n99026\t53065\tNine mile falls\tWA\tStevens County\tH1\n99114\t53065\tColville\tWA\tStevens County\tH1\n99173\t53065\tSpringdale\tWA\tStevens County\tH1\n99131\t53065\tGifford\tWA\tStevens County\tH1\n99148\t53065\tLoon lake\tWA\tStevens County\tH1\n99141\t53065\tKettle falls\tWA\tStevens County\tH1\n99167\t53065\tRice\tWA\tStevens County\tH1\n99151\t53065\tMarcus\tWA\tStevens County\tH1\n99122\t53065\tDavenport\tWA\tStevens County\tH1\n99101\t53065\tAddy\tWA\tStevens County\tH1\n99110\t53065\tClayton\tWA\tStevens County\tH1\n99137\t53065\tHunters\tWA\tStevens County\tH1\n99126\t53065\tEvans\tWA\tStevens County\tH1\n99160\t53065\tOrient\tWA\tStevens County\tH1\n99181\t53065\tValley\tWA\tStevens County\tH1\n99013\t53065\tFord\tWA\tStevens County\tH1\n99129\t53065\tFruitland\tWA\tStevens County\tH1\n99040\t53065\tWellpinit\tWA\tStevens County\tH1\n98505\t53067\tOlympia\tWA\tThurston County\tH1\n98501\t53067\tOlympia\tWA\tThurston County\tH1\n98506\t53067\tOlympia\tWA\tThurston County\tH1\n98512\t53067\tOlympia\tWA\tThurston County\tH1\n98530\t53067\tBucoda\tWA\tThurston County\tH1\n98597\t53067\tYelm\tWA\tThurston County\tH1\n98576\t53067\tRainier\tWA\tThurston County\tH1\n98509\t53067\tLacey\tWA\tThurston County\tH1\n98540\t53067\tEast olympia\tWA\tThurston County\tH1\n98502\t53067\tOlympia\tWA\tThurston County\tH1\n98507\t53067\tOlympia\tWA\tThurston County\tH1\n98579\t53067\tRochester\tWA\tThurston County\tH1\n98556\t53067\tLittlerock\tWA\tThurston County\tH1\n98531\t53067\tCentralia\tWA\tThurston County\tH1\n98508\t53067\tOlympia\tWA\tThurston County\tH1\n98568\t53067\tOakville\tWA\tThurston County\tH1\n98511\t53067\tTumwater\tWA\tThurston County\tH1\n98503\t53067\tLacey\tWA\tThurston County\tH1\n98513\t53067\tOlympia\tWA\tThurston County\tH1\n98589\t53067\tTenino\tWA\tThurston County\tH1\n98516\t53067\tOlympia\tWA\tThurston County\tH1\n98621\t53069\tGrays river\tWA\tWahkiakum County\tH1\n98647\t53069\tSkamokawa\tWA\tWahkiakum County\tH1\n98632\t53069\tLongview\tWA\tWahkiakum County\tH1\n98612\t53069\tCathlamet\tWA\tWahkiakum County\tH1\n98638\t53069\tNaselle\tWA\tWahkiakum County\tH1\n98643\t53069\tRosburg\tWA\tWahkiakum County\tH1\n99329\t53071\tDixie\tWA\tWalla Walla County\tH1\n99363\t53071\tWallula\tWA\tWalla Walla County\tH1\n99323\t53071\tBurbank\tWA\tWalla Walla County\tH1\n99328\t53071\tDayton\tWA\tWalla Walla County\tH1\n99361\t53071\tWaitsburg\tWA\tWalla Walla County\tH1\n99360\t53071\tTouchet\tWA\tWalla Walla County\tH1\n99324\t53071\tCollege place\tWA\tWalla Walla County\tH1\n99348\t53071\tPrescott\tWA\tWalla Walla County\tH1\n99362\t53071\tWalla walla\tWA\tWalla Walla County\tH1\n98266\t53073\tMaple falls\tWA\tWhatcom County\tH1\n98237\t53073\tConcrete\tWA\tWhatcom County\tH1\n98240\t53073\tCuster\tWA\tWhatcom County\tH1\n98225\t53073\tBellingham\tWA\tWhatcom County\tH1\n98276\t53073\tNooksack\tWA\tWhatcom County\tH1\n98264\t53073\tLynden\tWA\tWhatcom County\tH1\n98248\t53073\tFerndale\tWA\tWhatcom County\tH1\n98284\t53073\tSedro woolley\tWA\tWhatcom County\tH1\n98283\t53073\tRockport\tWA\tWhatcom County\tH1\n98231\t53073\tBlaine\tWA\tWhatcom County\tH1\n98295\t53073\tSumas\tWA\tWhatcom County\tH1\n98244\t53073\tDeming\tWA\tWhatcom County\tH1\n98230\t53073\tBlaine\tWA\tWhatcom County\tH1\n98227\t53073\tBellingham\tWA\tWhatcom County\tH1\n98228\t53073\tBellingham\tWA\tWhatcom County\tH1\n98220\t53073\tAcme\tWA\tWhatcom County\tH1\n98262\t53073\tLummi island\tWA\tWhatcom County\tH1\n98247\t53073\tEverson\tWA\tWhatcom County\tH1\n98281\t53073\tPoint roberts\tWA\tWhatcom County\tH1\n98229\t53073\tBellingham\tWA\tWhatcom County\tH1\n98226\t53073\tBellingham\tWA\tWhatcom County\tH1\n99170\t53075\tRosalia\tWA\tWhitman County\tH1\n99176\t53075\tThornton\tWA\tWhitman County\tH1\n99163\t53075\tPullman\tWA\tWhitman County\tH1\n99171\t53075\tSaint john\tWA\tWhitman County\tH1\n99033\t53075\tTekoa\tWA\tWhitman County\tH1\n99333\t53075\tHooper\tWA\tWhitman County\tH1\n99004\t53075\tCheney\tWA\tWhitman County\tH1\n99161\t53075\tPalouse\tWA\tWhitman County\tH1\n99125\t53075\tEndicott\tWA\tWhitman County\tH1\n99179\t53075\tUniontown\tWA\tWhitman County\tH1\n99136\t53075\tHay\tWA\tWhitman County\tH1\n99111\t53075\tColfax\tWA\tWhitman County\tH1\n99149\t53075\tMalden\tWA\tWhitman County\tH1\n99017\t53075\tLamont\tWA\tWhitman County\tH1\n99130\t53075\tGarfield\tWA\tWhitman County\tH1\n99164\t53075\tPullman\tWA\tWhitman County\tH1\n99128\t53075\tFarmington\tWA\tWhitman County\tH1\n99174\t53075\tSteptoe\tWA\tWhitman County\tH1\n99113\t53075\tColton\tWA\tWhitman County\tH1\n99158\t53075\tOakesdale\tWA\tWhitman County\tH1\n99403\t53075\tClarkston\tWA\tWhitman County\tH1\n99143\t53075\tLacrosse\tWA\tWhitman County\tH1\n99104\t53075\tBelmont\tWA\tWhitman County\tH1\n99102\t53075\tAlbion\tWA\tWhitman County\tH1\n98903\t53077\tYakima\tWA\tYakima County\tH1\n98907\t53077\tYakima\tWA\tYakima County\tH1\n98951\t53077\tWapato\tWA\tYakima County\tH1\n98936\t53077\tMoxee\tWA\tYakima County\tH1\n98923\t53077\tCowiche\tWA\tYakima County\tH1\n98952\t53077\tWhite swan\tWA\tYakima County\tH1\n98920\t53077\tBrownstown\tWA\tYakima County\tH1\n98942\t53077\tSelah\tWA\tYakima County\tH1\n99322\t53077\tBickleton\tWA\tYakima County\tH1\n98901\t53077\tYakima\tWA\tYakima County\tH1\n98908\t53077\tYakima\tWA\tYakima County\tH1\n98902\t53077\tYakima\tWA\tYakima County\tH1\n98939\t53077\tParker\tWA\tYakima County\tH1\n98944\t53077\tSunnyside\tWA\tYakima County\tH1\n98909\t53077\tYakima\tWA\tYakima County\tH1\n98953\t53077\tZillah\tWA\tYakima County\tH1\n99350\t53077\tProsser\tWA\tYakima County\tH1\n98947\t53077\tTieton\tWA\tYakima County\tH1\n98938\t53077\tOutlook\tWA\tYakima County\tH1\n98937\t53077\tNaches\tWA\tYakima County\tH1\n98935\t53077\tMabton\tWA\tYakima County\tH1\n98930\t53077\tGrandview\tWA\tYakima County\tH1\n98948\t53077\tToppenish\tWA\tYakima County\tH1\n98921\t53077\tBuena\tWA\tYakima County\tH1\n98932\t53077\tGranger\tWA\tYakima County\tH1\n98933\t53077\tHarrah\tWA\tYakima County\tH1\n26267\t54001\tEllamore\tWV\tBarbour County\tH1\n26275\t54001\tJunior\tWV\tBarbour County\tH1\n26330\t54001\tBridgeport\tWV\tBarbour County\tH1\n26416\t54001\tPhilippi\tWV\tBarbour County\tH1\n26354\t54001\tGrafton\tWV\tBarbour County\tH1\n26347\t54001\tFlemington\tWV\tBarbour County\tH1\n26250\t54001\tBelington\tWV\tBarbour County\tH1\n26349\t54001\tGalloway\tWV\tBarbour County\tH1\n26283\t54001\tMontrose\tWV\tBarbour County\tH1\n26201\t54001\tBuckhannon\tWV\tBarbour County\tH1\n26405\t54001\tMoatsville\tWV\tBarbour County\tH1\n26440\t54001\tThornton\tWV\tBarbour County\tH1\n26238\t54001\tVolga\tWV\tBarbour County\tH1\n25411\t54003\tBerkeley springs\tWV\tBerkeley County\tH1\n25420\t54003\tGerrardstown\tWV\tBerkeley County\tH1\n25401\t54003\tMartinsburg\tWV\tBerkeley County\tH1\n25413\t54003\tBunker hill\tWV\tBerkeley County\tH1\n25419\t54003\tFalling waters\tWV\tBerkeley County\tH1\n25402\t54003\tMartinsburg\tWV\tBerkeley County\tH1\n25443\t54003\tShepherdstown\tWV\tBerkeley County\tH1\n25427\t54003\tHedgesville\tWV\tBerkeley County\tH1\n25404\t54003\tMartinsburg\tWV\tBerkeley County\tH1\n25405\t54003\tMartinsburg\tWV\tBerkeley County\tH1\n25430\t54003\tKearneysville\tWV\tBerkeley County\tH1\n25403\t54003\tMartinsburg\tWV\tBerkeley County\tH1\n25428\t54003\tInwood\tWV\tBerkeley County\tH1\n25421\t54003\tGlengary\tWV\tBerkeley County\tH1\n25529\t54005\tJulian\tWV\tBoone County\tH1\n25209\t54005\tWhitesville\tWV\tBoone County\tH1\n25051\t54005\tCosta\tWV\tBoone County\tH1\n25206\t54005\tVan\tWV\tBoone County\tH1\n25053\t54005\tDanville\tWV\tBoone County\tH1\n25181\t54005\tSeth\tWV\tBoone County\tH1\n25114\t54005\tJeffrey\tWV\tBoone County\tH1\n25009\t54005\tAshford\tWV\tBoone County\tH1\n25508\t54005\tChapmanville\tWV\tBoone County\tH1\n25081\t54005\tFoster\tWV\tBoone County\tH1\n25208\t54005\tWharton\tWV\tBoone County\tH1\n25154\t54005\tPeytona\tWV\tBoone County\tH1\n25049\t54005\tComfort\tWV\tBoone County\tH1\n25130\t54005\tMadison\tWV\tBoone County\tH1\n25108\t54005\tHewett\tWV\tBoone County\tH1\n25148\t54005\tOrgas\tWV\tBoone County\tH1\n25142\t54005\tNellis\tWV\tBoone County\tH1\n25169\t54005\tRidgeview\tWV\tBoone County\tH1\n25024\t54005\tBloomingrose\tWV\tBoone County\tH1\n25093\t54005\tGordon\tWV\tBoone County\tH1\n25149\t54005\tOttawa\tWV\tBoone County\tH1\n25165\t54005\tRacine\tWV\tBoone County\tH1\n25205\t54005\tUneeda\tWV\tBoone County\tH1\n25204\t54005\tTwilight\tWV\tBoone County\tH1\n25193\t54005\tSylvester\tWV\tBoone County\tH1\n25028\t54005\tBob white\tWV\tBoone County\tH1\n25203\t54005\tTurtle creek\tWV\tBoone County\tH1\n25021\t54005\tBim\tWV\tBoone County\tH1\n26412\t54007\tOrlando\tWV\tBraxton County\tH1\n26601\t54007\tSutton\tWV\tBraxton County\tH1\n26203\t54007\tErbacon\tWV\tBraxton County\tH1\n26619\t54007\tExchange\tWV\tBraxton County\tH1\n26376\t54007\tIreland\tWV\tBraxton County\tH1\n26627\t54007\tHeaters\tWV\tBraxton County\tH1\n26621\t54007\tFlatwoods\tWV\tBraxton County\tH1\n26335\t54007\tBurnsville\tWV\tBraxton County\tH1\n26447\t54007\tWalkersville\tWV\tBraxton County\tH1\n26623\t54007\tFrametown\tWV\tBraxton County\tH1\n26624\t54007\tGassaway\tWV\tBraxton County\tH1\n26611\t54007\tCedarville\tWV\tBraxton County\tH1\n26636\t54007\tRosedale\tWV\tBraxton County\tH1\n26629\t54007\tLittle birch\tWV\tBraxton County\tH1\n25063\t54007\tDuck\tWV\tBraxton County\tH1\n26631\t54007\tNapier\tWV\tBraxton County\tH1\n26222\t54007\tHacker valley\tWV\tBraxton County\tH1\n26615\t54007\tCopen\tWV\tBraxton County\tH1\n26070\t54009\tWellsburg\tWV\tBrooke 
